vi "DFD Plot NStage MRate Freq Response.vi"(5 "output option":u16(ring) items=["Auto", "Floating-Point Only", "Fixed-Point Only"], 6 "fs in [Hz]":dbl=-1.0 format="%.2f", 7 "# freq bins":i32=-1, 8 "error in (no error)":errorcluster, 9 "dB on? (T)":bool=TRUE, 10 "phase view":T6, 11 "multirate filters in":T1[](array[typedef]) {"mMRate_SumWl" min=1 max=32 step=1; "mMRate_InputIwl" min=1 max=32 step=1; "mMRate_GainWl" min=1 max=32 step=1; "mMRate_OutputWl" min=1 max=32 step=1; "mMRate_InputWl" min=1 max=32 step=1; "mMRate_CoefWl" min=1 max=32 step=1; "mMRate_Mode" items=["Default"=-1, "No Rate Change"=0, "Interpolation"=1, "Decimation"=2, "Interpolated"=3, "Rational"=4]}) -> (0 "error out":errorcluster, 1 "phase responses":cluster{"f0":dbl, "df":dbl, "values":dbl[]}[](graph), 2 "magnitude responses":cluster{"f0":dbl, "df":dbl, "values":dbl[]}[](graph), 3 "multirate filters out":T1[](array[typedef]) {"mMRate_SumWl" min=1 max=32 step=1; "mMRate_InputIwl" min=1 max=32 step=1; "mMRate_GainWl" min=1 max=32 step=1; "mMRate_OutputWl" min=1 max=32 step=1; "mMRate_InputWl" min=1 max=32 step=1; "mMRate_CoefWl" min=1 max=32 step=1; "mMRate_Mode" items=["Default"=-1, "No Rate Change"=0, "Interpolation"=1, "Decimation"=2, "Interpolated"=3, "Rational"=4]})   [LabVIEW 2017, in "NI_DigFilterLicensed.lvlib"]
doc: "Plots the frequency responses, including the magnitude and phase responses, of a multistage multirate filter."
uses:
  <vilib>/addons/Digital Filter Design/NI_DigFilterLicensed.lvlib
  <vilib>/addons/Digital Filter Design/_Objects.llb/DFD Multirate Filter Obj.ctl
  <vilib>/addons/Digital Filter Design/_Objects.llb/DFD Multirate Mode.ctl
  <vilib>/addons/Digital Filter Design/_Objects.llb/DFD Coef Norm Type.ctl
  <vilib>/addons/Digital Filter Design/_Objects.llb/DFD Round-off Mode.ctl
  <vilib>/addons/Digital Filter Design/_Objects.llb/DFD FXP MRate Multiply Mode.ctl
  <vilib>/addons/Digital Filter Design/_Objects.llb/DFD Phase Setting.ctl
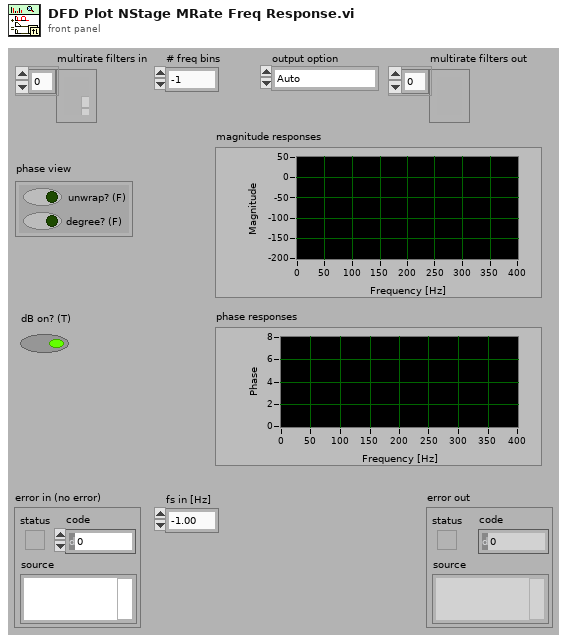
[diagram p1: front panel]
types:
  T1 = typedef "NI_DigFilterLicensed.lvlib/DFD Multirate Filter Obj.ctl" = cluster{"mMRate_Structure":enum16{"CIC", "FIR", "IIR", "Lattice"}, "mMRate_Mode":T2, "mMRate_Factor":i32, "mMRate_FIRParams":cluster{"mMRate_FIR_H":dbl[], "mMRate_FIR_IsNyquist?":bool, "mMRate_FIR_IsSymmetric?":bool}, "mMRate_CICParams":cluster{"mMRate_CIC_#Stage":i32, "mMRate_CIC_Lag":i32, "mMRate_CIC_Type":enum16{"Lowpass", "Highpass"}}, "mMRate_Order":i32, "mMRate_Version":string, "mMRate_Comments":string, "mMRate_RationalFactor":cluster{"mMRate_L":i32, "mMRate_M":i32}, "mMRate_Fs":dbl, "mMRate_Quantized?":bool, "mMRate_QFilterGain":dbl, "mMRate_CoefWl":i16, "mMRate_Scaling":cluster{"mMRate_ScaleByPowerOf2?":bool, "mMRate_ScaleType":T3}, "mMRate_InputWl":i16, "mMRate_OutputWl":i16, "mMRate_OutputMode":T4, "mMRate_MultMode":T5, "mMRate_BitPruning":bool, "mMRate_GainWl":i16, "mMRate_OutputFwl":i16, "mMRate_SumIwl":i16, "mMRate_InputIwl ":i16, "mMRate_SumWl":i16, "mMRate_CoefIwl":i16}
  T2 = typedef "NI_DigFilterLicensed.lvlib/DFD Multirate Mode.ctl" = i16
  T3 = typedef "NI_DigFilterLicensed.lvlib/DFD Coef Norm Type.ctl" = enum16{"No Norm", "Time Domain 1-Norm", "Time Domain 2-Norm", "Time Domain Inf-Norm"}
  T4 = typedef "NI_DigFilterLicensed.lvlib/DFD Round-off Mode.ctl" = enum16{"Nearest", "Truncation"}
  T5 = typedef "NI_DigFilterLicensed.lvlib/DFD FXP MRate Multiply Mode.ctl" = enum16{"Truncated", "Full"}
  T6 = typedef "NI_DigFilterLicensed.lvlib/DFD Phase Setting.ctl" = cluster{"unwrap? (F)":bool, "degree? (F)":bool}
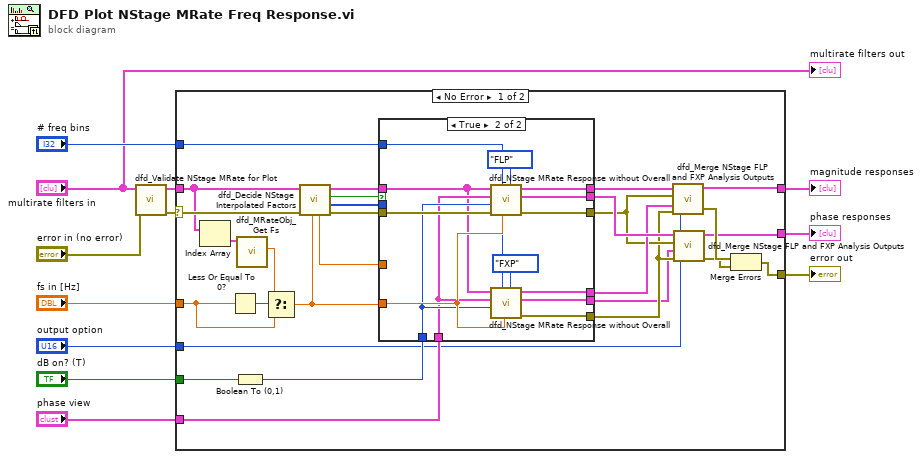
[diagram p0: block diagram]
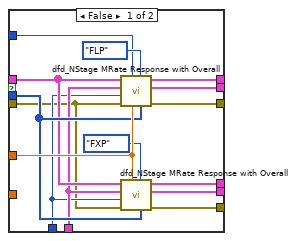
[diagram p2: hidden frame]
diagram:
  n1 = call <vilib>:"dfd_Validate NStage MRate for Plot.vi"("error in (no error)"="error in (no error)", "multirate filters in"="multirate filters in") -> ("error out"=w2:errorcluster, "multirate filters out"=w4:T1[])  [unwired: 8 out]
  n2 = case shown="No Error" w2 {
    selector: w2 -> [w28 w70]
    tunnel: w4 -> [w27 _]
    tunnel: "fs in [Hz]" -> [w39 _]
    tunnel: "dB on? (T)" -> [w38 _]
    tunnel: "phase view" -> [w37 _]
    tunnel: [w16 w70] -> w9
    tunnel: [w14 _] -> w8
    tunnel: [w15 _] -> w7
    tunnel: "# freq bins" -> [w36 _]
    tunnel: "output option" -> [w13 _]
    frame No Error {
      n3 = Index Array(array=w27) -> (element=w26:T1)  [unwired: 1 in]
      n4 = Less Or Equal To 0?(x=w39) -> (x <= 0?=w40:bool)
      n5 = Boolean To (0,1)(Boolean=w38) -> (0, 1=w35:i16)
      n6 = call <vilib>:"dfd_MRateObj_Get Fs.vi"("multirate filter in"=w26) -> ("fs"=w25:dbl)  [unwired: 10 out]
      n7 = Select(t=w25, s=w40, f=w39) -> (s? t:f=w29:dbl)
      n8 = call <vilib>:"dfd_Decide NStage Interpolated Factors.vi"("fs in [Hz]"=w29, "error in (no error)"=w28, "multirate filters in"=w27) -> ("error out"=w31:errorcluster, "interpolated factors"=w32:i32[], "no overall?"=w33:bool, "dup multirate filters in"=w34:T1[], "equivalent fs"=w30:dbl)  [unwired: 1 in, 3 out]
      n9 = case shown="True" w33 {
        tunnel: w37 -> [w49 w62]
        tunnel: w36 -> [w52 w59]
        tunnel: w35 -> [w48 w63]
        tunnel: w29 -> [_ w64]
        tunnel: w34 -> [w50 w61]
        tunnel: w32 -> [w53 _]
        tunnel: w31 -> [w47 w69]
        tunnel: w30 -> [w54 _]
        tunnel: [w46 w66] -> w22
        tunnel: [w45 w65] -> w21
        tunnel: [w44 w58] -> w20
        tunnel: [w43 w57] -> w17
        tunnel: [w42 w67] -> w19
        tunnel: [w41 w56] -> w18
        frame False {
          n10 = call <vilib>:"dfd_NStage MRate Response with Overall.vi"("interpolated factors"=w53, "type (FLP)"=enum16{"FLP", "FXP"}."FLP", "fs [Hz]"=w54, "# freq bins (auto)"=w52, "error in (no error)"=w47, "magnitude"=w48, "phase view"=w49, "multirate filters in"=w50) -> ("error out"=w42:errorcluster, "phase"=w45:cluster{dbl, "df":dbl, "phase":dbl[]}[], "mag"=w46:cluster{dbl, "df":dbl, "magnitude":dbl[]}[])  [unwired: 1 out]
          n11 = call <vilib>:"dfd_NStage MRate Response with Overall.vi"("interpolated factors"=w53, "type (FLP)"=enum16{"FLP", "FXP"}."FXP", "fs [Hz]"=w54, "# freq bins (auto)"=w52, "error in (no error)"=w47, "magnitude"=w48, "phase view"=w49, "multirate filters in"=w50) -> ("error out"=w41:errorcluster, "phase"=w43:cluster{dbl, "df":dbl, "phase":dbl[]}[], "mag"=w44:cluster{dbl, "df":dbl, "magnitude":dbl[]}[])  [unwired: 1 out]
        }
        frame True {
          n12 = call <vilib>:"dfd_NStage MRate Response without Overall.vi"("type (FLP)"=enum16{"FLP", "FXP"}."FLP", "fs [Hz]"=w64, "# freq bins (auto)"=w59, "error in (no error)"=w69, "magnitude"=w63, "phase view"=w62, "multirate filters in"=w61) -> ("error out"=w67:errorcluster, "phase"=w65:cluster{dbl, "df":dbl, "phase":dbl[]}[], "mag"=w66:cluster{dbl, "df":dbl, "magnitude":dbl[]}[])  [unwired: 2 out]
          n13 = call <vilib>:"dfd_NStage MRate Response without Overall.vi"("type (FLP)"=enum16{"FLP", "FXP"}."FXP", "fs [Hz]"=w64, "# freq bins (auto)"=w59, "magnitude"=w63, "phase view"=w62, "multirate filters in"=w61) -> ("error out"=w56:errorcluster, "phase"=w57:cluster{dbl, "df":dbl, "phase":dbl[]}[], "mag"=w58:cluster{dbl, "df":dbl, "magnitude":dbl[]}[])  [unwired: 1 in, 2 out]
        }
      }
      n14 = call <vilib>:"dfd_Merge NStage FLP and FXP Analysis Outputs.vi"("output option"=w13, "error in FXP"=w18, 9:"freq response"=w20, "error in FLP"=w19, 11:"freq response"=w22) -> ("error out"=w24:errorcluster, "freq response"=w14:cluster{"f0":dbl, "df":dbl, "values":dbl[]}[])  [unwired: 5 out]
      n15 = call <vilib>:"dfd_Merge NStage FLP and FXP Analysis Outputs.vi"("output option"=w13, "error in FXP"=w18, 9:"freq response"=w17, "error in FLP"=w19, 11:"freq response"=w21) -> ("error out"=w23:errorcluster, "freq response"=w15:cluster{"f0":dbl, "df":dbl, "values":dbl[]}[])  [unwired: 5 out]
      n16 = Merge Errors(w24, w23) -> (w16:errorcluster)
    }
    frame Error {
    }
  }
  "error out" <- w9
  "magnitude responses" <- w8
  "phase responses" <- w7
  "multirate filters out" <- "multirate filters in"
